vi "Build RT Data Cluster.vi"(8 "error in (no error)":errorcluster, 10 "Compiled Settings Parameters":variant, 11 "Process In":refnum<class "Process.lvclass">) -> (0 "error out":errorcluster, 2 "RT State Variables":T1 {"Settings"."Tx Packet Info"."Endianness" items=["big-endian"=0, "little-indian"=2]; "Settings"."Rx Packet Info"."Endianness" items=["big-endian"=0, "little-indian"=2]}, 3 "Process Out":refnum<class "Process.lvclass">)   [LabVIEW 2016]
uses:
  <vilib>/NI/NIVS Inline Async API/_VS Inline Async API/Process/Process.lvclass
  RTStateVariables.ctl
  <vilib>/NI/NIVS Inline Async API/_VS Inline Async API/VS Inline Async API/VS Inline Async API.lvclass
  Shared/Compiled.Settings.ctl
  Shared/Rx.PacketInfo.ctl
  System Explorer/Types/Channel Data Type.ctl
  Shared/Tx.PacketInfo.ctl
  <vilib>/NI/NIVS Inline Async API/_Data Access Engine/Data Access Engine/Types/Write.DVR.ctl
  <vilib>/NI/NIVS Inline Async API/_Data Access Engine/Access Type Classes/Write/Write.lvclass
  <vilib>/NI/NIVS Inline Async API/_Data Access Engine/Data Access Engine/Types/Read.DVR.ctl
  <vilib>/NI/NIVS Inline Async API/_Data Access Engine/Access Type Classes/Read/Read.lvclass
  <vilib>/NI/NIVS Inline Async API/_VS Inline Async API/Process/Process.lvclass/Process.ctl
  <vilib>/NI/NIVS Inline Async API/_VS Inline Async API/Process/Data Member Access/Read Data Access.vi
  <vilib>/NI/NIVS Inline Async API/_Data Access Engine/Data Access Engine/Methods/Write.Lookup.vi
  <vilib>/NI/NIVS Inline Async API/_Data Access Engine/Data Access Engine/Methods/Read.Lookup.vi
  <vilib>/NI/NIVS Inline Async API/_Data Access Engine/Data Access Engine/Data Access Engine.lvclass
  Shared/UDP-Custom-Device Shared.lvlib
  UDP-Custom-Device Engine.lvlib
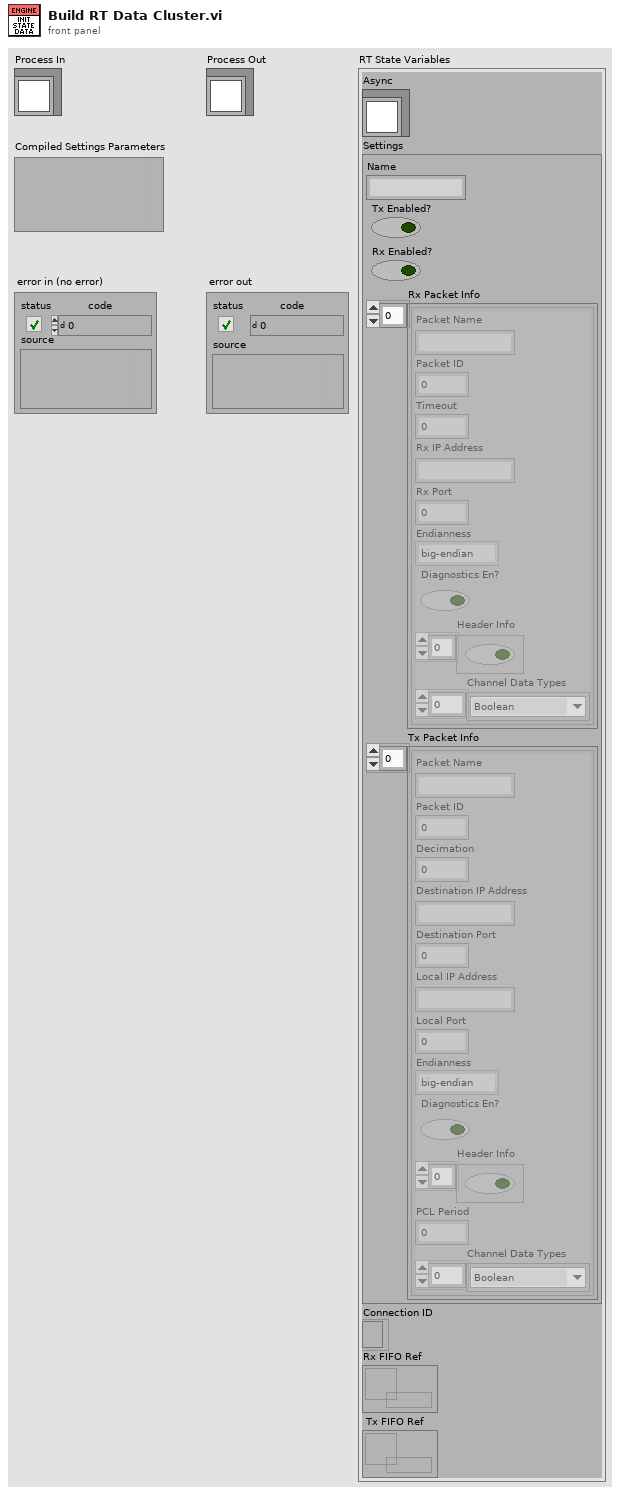
[diagram p1: front panel]
types:
  T1 = typedef "UDP-Custom-Device Engine.lvlib/RTStateVariables.ctl" = cluster{"Async":refnum<class "VS Inline Async API.lvclass">, "Settings":T2, "Connection ID":refnum<k16>, "Rx FIFO Ref":T6, "Tx FIFO Ref":T7}
  T2 = typedef "UDP-Custom-Device Shared.lvlib/Compiled.Settings.ctl" = cluster{"Name":string, "Tx Enabled?":bool, "Rx Enabled?":bool, "Rx Packet Info":T3[], "Tx Packet Info":T5[]}
  T3 = typedef "UDP-Custom-Device Shared.lvlib/Rx.PacketInfo.ctl" = cluster{"Packet Name":string, "Packet ID":i32, "Timeout":i32, "Rx IP Address":string, "Rx Port":i32, "Endianness":u16, "Diagnostics En?":bool, "Header Info":bool[], "Channel Data Types":T4[]}
  T4 = typedef "UDP-Custom-Device Shared.lvlib/Channel Data Type.ctl" = enum16{"Boolean", "Single"}
  T5 = typedef "UDP-Custom-Device Shared.lvlib/Tx.PacketInfo.ctl" = cluster{"Packet Name":string, "Packet ID":i32, "Decimation":i32, "Destination IP Address":string, "Destination Port":i32, "Local IP Address":string, "Local Port":i32, "Endianness":u16, "Diagnostics En?":bool, "Header Info":bool[], "PCL Period":u32, "Channel Data Types":T4[]}
  T6 = typedef "Data Access Engine.lvlib/Data Access Engine.lvclass/Write.DVR.ctl" = refnum<data-value>
  T7 = typedef "Data Access Engine.lvlib/Data Access Engine.lvclass/Read.DVR.ctl" = refnum<data-value>
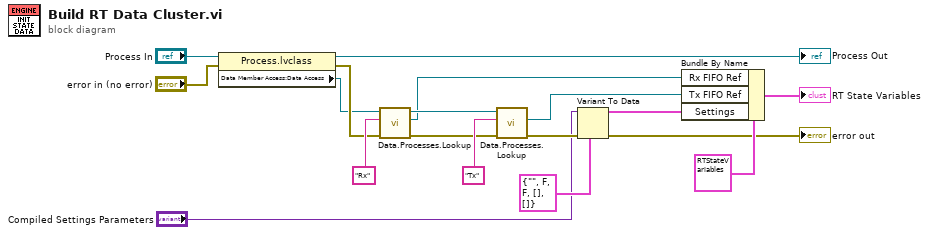
[diagram p0: block diagram]
diagram:
  n1 = property class="Process.lvclass"(reference="Process In", error in="error in (no error)") -> (reference out=→"Process Out":refnum<class "Process.lvclass">, error out=w14:errorcluster, "Data Member Access:Data Access"=w10:refnum<class "Data Access Engine.lvclass">)
  n2 = call-poly <vilib>:"Data.Processes.Lookup.vi"("error in (no error)"=w14, "Name"="Rx", "Data Access API in"=w10) -> ("error out"=w16:errorcluster, "Ref"=w1:T6, "Data Access API out"=w15:refnum<class "Data Access Engine.lvclass">)  [unwired: 5 in, 1 out]
  n3 = call-poly <vilib>:"Data.Processes.Lookup.vi"("error in (no error)"=w16, "Name"="Tx", "Data Access API in"=w15) -> ("error out"=w8:errorcluster, "Ref"=w2:T7)  [unwired: 5 in, 2 out]
  n4 = Variant To Data(error in=w8, type=T2 {"Name"="", "Tx Enabled?"=FALSE, "Rx Enabled?"=FALSE, "Rx Packet Info"=[], "Tx Packet Info"=[]} ("Compiled.Settings"), Variant="Compiled Settings Parameters") -> (data=w5:T2, error out=→"error out":errorcluster)
  n5 = Bundle By Name(cluster=T1 {"Async"=refnum, "Settings"={"Name"="", "Tx Enabled?"=FALSE, "Rx Enabled?"=FALSE, "Rx Packet Info"=[], "Tx Packet Info"=[]}, "Connection ID"=refnum, "Rx FIFO Ref"=refnum, "Tx FIFO Ref"=refnum} ("RT State Variables"), "Rx FIFO Ref"=w1, "Tx FIFO Ref"=w2, "Settings"=w5) -> (→"RT State Variables":T1)
